vi "Trigger.vi"(1 "触发电平":dbl, 2 "触发参数设置":cluster{"枚举":T1, "触发基准电平":dbl}) -> (0 "Trigger？":bool)   [LabVIEW 2018]
uses:
  Ctl/TriggerType.ctl
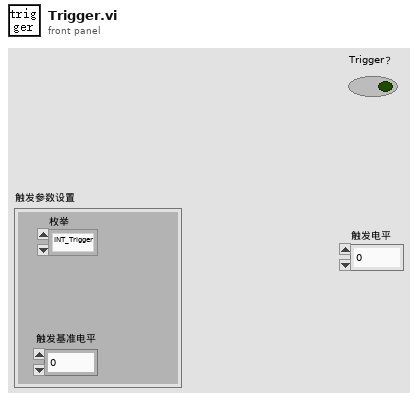
[diagram p1: front panel]
types:
  T1 = typedef "TriggerType.ctl" = enum16{"INT_Trigger", "Ext_Trigger"}
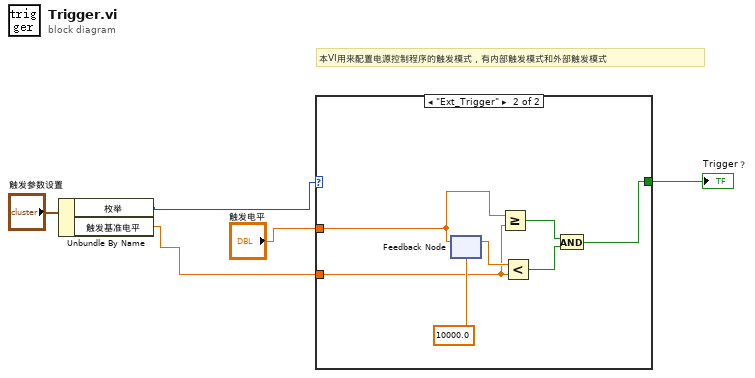
[diagram p0: block diagram]
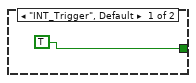
[diagram p2: hidden frame]
diagram:
  # "本VI用来配置电源控制程序的触发模式，有内部触发模式和外部触发模式"
  n1 = Unbundle By Name("触发参数设置") -> ("枚举"=w3:T1, "触发基准电平"=w2:dbl)
  n2 = case shown="\"Ext_Trigger\"" w3 {
    tunnel: [TRUE w10] -> w5
    tunnel: "触发电平" -> [_ w7]
    tunnel: w2 -> [_ w8]
    frame "INT_Trigger", Default {
    }
    frame "Ext_Trigger" {
      n3 = feedback-in #1(w7) -> ()
      n4 = feedback #1(10000.0 ("触发电平")) -> (w13:dbl)
      n5 = Greater Or Equal?(x=w7, y=w8) -> (x >= y?=w12:bool)
      n6 = Less?(x=w13, y=w8) -> (x < y?=w11:bool)
      n7 = And(x=w12, y=w11) -> (x .and. y?=w10:bool)
    }
  }
  "Trigger？" <- w5
